vi "Generate Data.vi"(8 "错误输入":cluster{"状态":bool, "代码":i32, "源":string}, 11 "通道数":i32) -> (0 "错误输出":cluster{"状态":bool, "代码":i32, "源":string}, 2 "功率谱":waveform(dbl)[](graph), 3 "时间数据":waveform(dbl)[](graph))   [LabVIEW 2012]
uses:
  Instance           3 21Saved   Generate Data .vi
  Instance           4 21Saved   Generate Data .vi
  <vilib>/express/express analysis/Spectral/Block/exnSpectralBlock spectral measurements power poly.vi
  <vilib>/express/express analysis/Spectral/Block/exnSpectralBlock spectral measurements power DDT.vi
  <vilib>/express/express analysis/Spectral/XNode/ExpressSpectralMeasurementsBlockNode.xnode
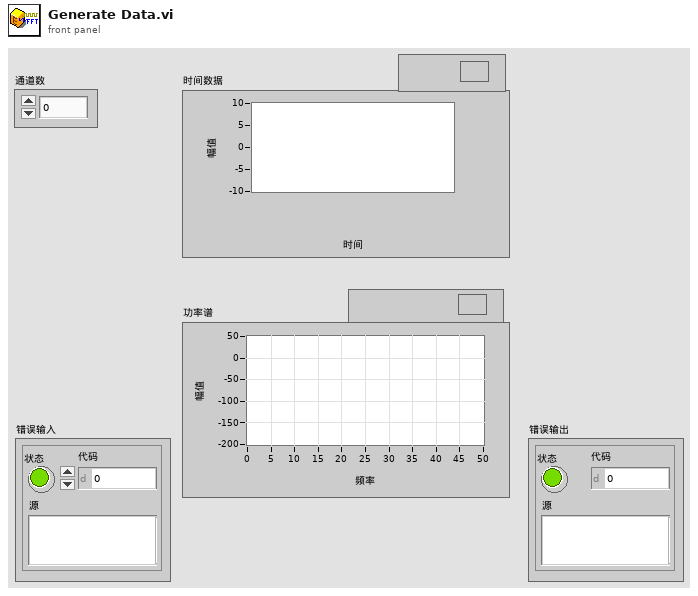
[diagram p1: front panel]
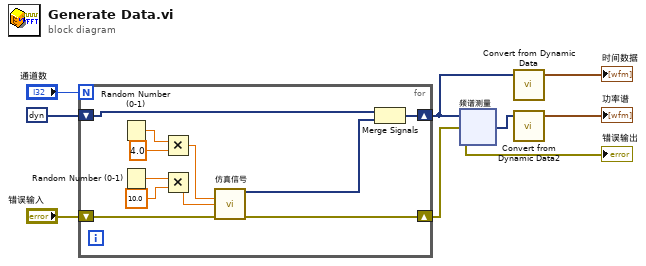
[diagram p0: block diagram]
diagram:
  n1 = for {
    N: "通道数" -> [_]
    shift-right: [w14] -> w4
    shift-left: "错误输入" -> [w18]
    shift-right: [w17] -> w2
    shift-left: dynamicdata [] ("空") -> [w15]
    n2 = Random Number (0-1) ("随机数(0-1)")() -> (number: 0 to 1=w12:dbl)
    n3 = Random Number (0-1) ("随机数(0-1)")() -> (number: 0 to 1=w20:dbl)
    n4 = Multiply ("乘")(x=w12, y=4.0) -> (x*y=w10:dbl)
    n5 = Multiply ("乘")(x=w20, y=10.0) -> (x*y=w11:dbl)
    n6 = call "仿真信号"("Frequency"=w10, "Amplitude"=w11, "error in (no error)"=w18) -> ("正弦"=w16:dynamicdata, "error out"=w14:errorcluster)  [unwired: 11 in]
    n7 = Merge Signals ("合并信号")(w15, w16) -> (w17:dynamicdata)
  }
  n8 = xnode "频谱测量"("信号"=w2, "错误输入（无错误）"=w4) -> ("功率谱"=w1:dynamicdata, "错误输出"=→"错误输出":errorcluster)
  n9 = call "Convert from Dynamic Data"("Dynamic Data Type"=w2) -> ("Array of Waveform"=→"时间数据":waveform(dbl)[])  [unwired: 3 in]
  n10 = call "Convert from Dynamic Data2"("Dynamic Data Type"=w1) -> ("Array of Waveform"=→"功率谱":waveform(dbl)[])  [unwired: 3 in]
